vi "生成-累积剂量报警记录数据文件-网络版.vi"(11 "探测器信息":T1) -> ()   [LabVIEW 2017]
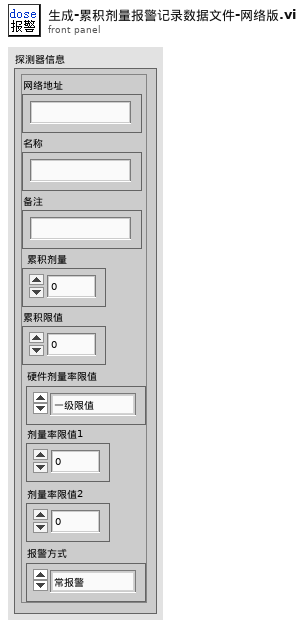
[diagram p1: front panel]
types:
  T1 = typedef "探测器信息.ctl" = cluster{"网络地址":string, "名称":string, "备注":string, "累积剂量":dbl, "累积限值":dbl, "硬件剂量率限值":T2, "剂量率限值1":dbl, "剂量率限值2":dbl, "报警方式":T3}
  T2 = typedef "探头剂量率限值选择.ctl" = enum16{"一级限值", "二级限值"}
  T3 = typedef "报警方式选择.ctl" = enum16{"常报警", "自动静音", "手动静音"}
  T4 = cluster{"起始时间":timestamp, "数值(rate/dose)":dbl, "报警累积":dbl}
  T5 = typedef "探头状态.ctl" = enum16{"正常", "离线", "禁用", "一级报警", "二级报警", "累积报警"}
  T6 = typedef "通用报警记录.ctl" = cluster{"探头状态":T5, "探头地址与信息":T1, "缓存绘图数据":T7, "平均值":dbl, "报警时长":cluster{"分":u16, "秒":u16}, "结论":string}
  T7 = typedef "时值缓存压缩模块.lvlib/缓存数据.ctl" = cluster{"时间":timestamp[], "数值":dbl[], "压缩等级数量":i32[], "最大值":cluster{"时间":timestamp, "数值":dbl}, "起始点":cluster{"时间":timestamp, "数值":dbl}, "容量限值":i32, "报警累积":dbl}
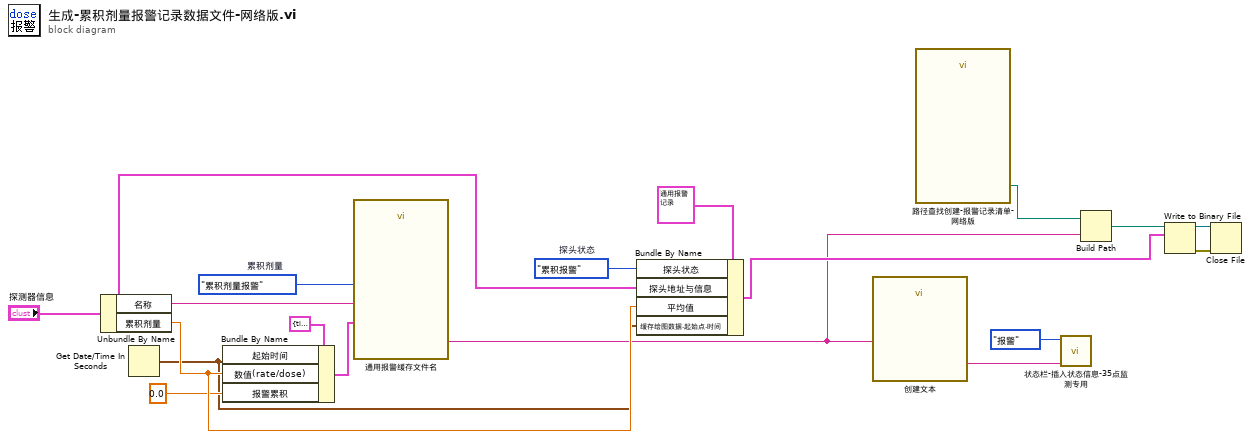
[diagram p0: block diagram]
diagram:
  w14 = enum16{"剂量率报警", "累积剂量报警"}."累积剂量报警"  # 累积剂量
  w17 = 探头状态."累积报警"  # 探头状态
  n1 = Unbundle By Name("探测器信息") -> ("名称"=w15:string, "累积剂量"=w12:dbl)
  n2 = Get Date/Time In Seconds() -> (seconds since 1Jan1904=w1:timestamp)
  n3 = Bundle By Name(cluster=T4 {"起始时间"=timestamp(0 s since 1904-01-01), "数值(rate/dose)"=0.0, "报警累积"=0.0} ("时值"), "起始时间"=w1, "数值(rate/dose)"=w12, "报警累积"=0.0 ("累积剂量")) -> (w16:T4)
  n4 = call "通用报警缓存文件名.vi"("报警类型"=w14, "时值"=w16, "名称"=w15) -> ("文件名"=w4:string)  [unwired: 8 in]
  n5 = Bundle By Name(cluster=T6 {"探头状态"=enum."正常", "探头地址与信息"={"网络地址"="", "名称"="", "备注"="", "累积剂量"=0.0, "累积限值"=0.0, "硬件剂量率限值"=enum."一级限值", "剂量率限值1"=0.0, "剂量率限值2"=0.0, "报警方式"=enum."常报警"}, "缓存绘图数据"={"时间"=[], "数值"=[], "压缩等级数量"=[], "最大值"={"时间"=timestamp(0 s since 1904-01-01), "数值"=0.0}, "起始点"={"时间"=timestamp(0 s since 1904-01-01), "数值"=0.0}, "容量限值"=0, "报警累积"=0.0}, "平均值"=0.0, "报警时长"={"分"=0, "秒"=0}, "结论"=""} ("报警记录"), "探头状态"=w17, "探头地址与信息"="探测器信息", "平均值"=w12, "缓存绘图数据.起始点.时间"=w1) -> (w8:T6)
  n6 = call "创建文本"("文件名"=w4) -> ("Result"=w9:string)  [unwired: 13 in, 1 out]
  n7 = call "路径查找创建-报警记录清单-网络版.vi"() -> ("缓存数据文件夹"=w11:path)  [unwired: 2 in, 13 out]
  n8 = call "状态栏-插入状态信息-35点监测专用.vi"("消息内容"=w9, "状态类型"=enum16{"全部", "报警", "通信", "设置"}."报警") -> ()  [unwired: 10 in]
  n9 = Build Path(base path=w11, name or relative path=w4) -> (appended path=w5:path)
  n10 = Write to Binary File(file (use dialog)=w5, data=w8) -> (refnum out=w6:refnum<file>, error out=w7:errorcluster)  [unwired: 4 in, 1 out]
  n11 = Close File(refnum=w6, error in=w7) -> ()  [unwired: 2 out]
